vi "clase5.vi"() -> ()   [LabVIEW 2011]
panel:
  out "A/C":bool
  out "Numero de Personas":i32
  out "Temperatura":i32(slide) scale=0.0..60.0
  in  "Seleccionar local":u16(ring) items=["Local1", "Local2", "local3"]
  # "Debemos seleccionar el local, luego generar el numero de personas entre 1-50 \ny la temperatura entre 1-60.\nEl A/C se enciende de acuerdo a los siguientes casos:\n\n\nLocal      Condicion para encender el A/C\nLocal1  Si la temperatura es mayor a 25 o el numero de empleados es mayor a 30 \nLocal2  Si la temperatura es mayor a 28 o el numero de empleados es mayor a 35 \nLocal3  Si la temperatura es mayor a 24 o el numero de empleados es mayor a 20"
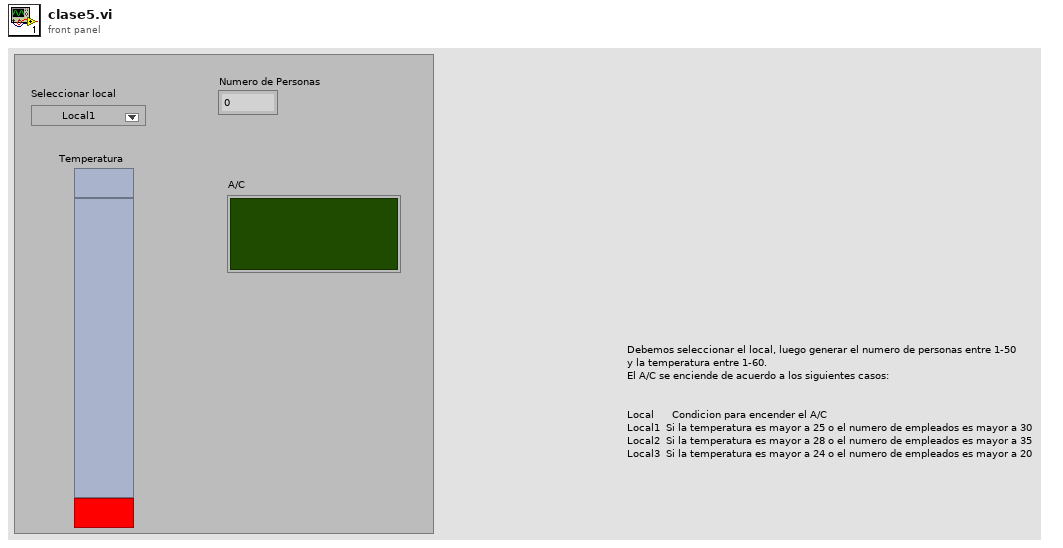
[diagram p1: front panel]
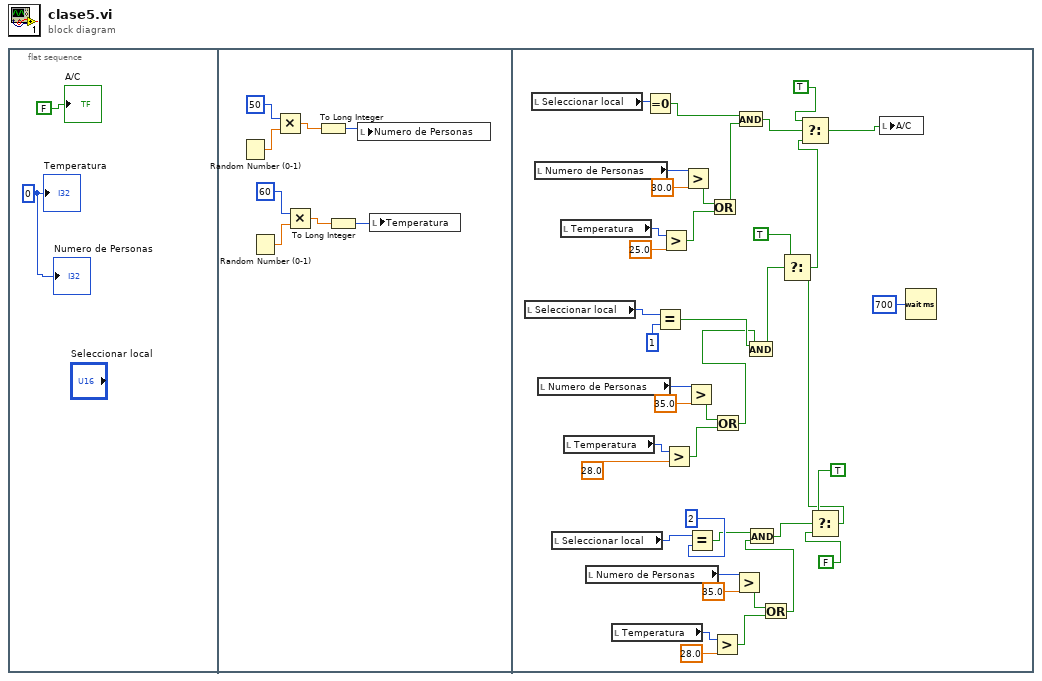
[diagram p0: block diagram]
diagram:
  n1 = flat-sequence {
    frame #0 {
      w1 = 0
      "Temperatura" <- w1
      "Numero de Personas" <- w1
      "A/C" <- FALSE
    }
    frame #1 {
      n2 = Random Number (0-1)() -> (number: 0 to 1=w9:dbl)
      n3 = Random Number (0-1)() -> (number: 0 to 1=w5:dbl)
      n4 = Multiply(x=50, y=w9) -> (x*y=w8:dbl)
      n5 = Multiply(x=60, y=w5) -> (x*y=w6:dbl)
      n6 = To Long Integer(number=w8) -> (32bit integer=w7:i32)
      n7 = To Long Integer(number=w6) -> (32bit integer=w3:i32)
      n8 = local write "Numero de Personas"(w7) -> ()
      n9 = local write "Temperatura"(w3) -> ()
    }
    frame #2 {
      n10 = local read "Seleccionar local"() -> (w21:u16)
      n11 = local read "Seleccionar local"() -> (w50:u16)
      n12 = local read "Numero de Personas"() -> (w48:i32)
      n13 = local read "Numero de Personas"() -> (w34:i32)
      n14 = local read "Seleccionar local"() -> (w17:u16)
      n15 = local read "Temperatura"() -> (w46:i32)
      n16 = local read "Temperatura"() -> (w36:i32)
      n17 = local read "Numero de Personas"() -> (w29:i32)
      n18 = local read "Temperatura"() -> (w27:i32)
      n19 = Equal To 0?(x=w50) -> (x = 0?=w43:bool)
      n20 = Equal?(x=w21, y=1) -> (x = y?=w20:bool)
      n21 = Greater?(x=w46, y=25.0) -> (0:w45:bool)
      n22 = Greater?(x=w36, y=28.0) -> (0:w37:bool)
      n23 = Greater?(x=w48, y=30.0) -> (0:w44:bool)
      n24 = Greater?(x=w34, y=35.0) -> (0:w38:bool)
      n25 = Equal?(x=w17, y=2) -> (x = y?=w15:bool)
      n26 = Or(x=w44, y=w45) -> (x .or. y?=w42:bool)
      n27 = Greater?(x=w27, y=28.0) -> (0:w26:bool)
      n28 = Or(x=w38, y=w37) -> (x .or. y?=w19:bool)
      n29 = Greater?(x=w29, y=35.0) -> (0:w25:bool)
      n30 = And(x=w43, y=w42) -> (x .and. y?=w41:bool)
      n31 = And(x=w20, y=w19) -> (x .and. y?=w18:bool)
      n32 = Or(x=w25, y=w26) -> (x .or. y?=w14:bool)
      n33 = And(x=w15, y=w14) -> (x .and. y?=w13:bool)
      n34 = Select(t=TRUE, s=w13, f=FALSE) -> (s? t:f=w23:bool)
      n35 = Select(t=TRUE, s=w18, f=w23) -> (s? t:f=w32:bool)
      n36 = Select(t=TRUE, s=w41, f=w32) -> (s? t:f=w39:bool)
      n37 = local write "A/C"(w39) -> ()
      n38 = Wait (ms)(milliseconds to wait=u32 700) -> ()  [unwired: 1 out]
    }
  }
